vi "Path Notation to Array.vi"(11 "Item Path":string) -> (3 "Nested Item Names":string[](array[string]))   [LabVIEW 2013, in "JSONtext.lvlib"]
uses:
  JSONtext.lvlib
  support/JSONtext support.lvlib
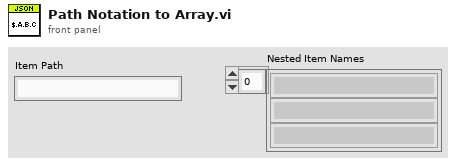
[diagram p1: front panel]
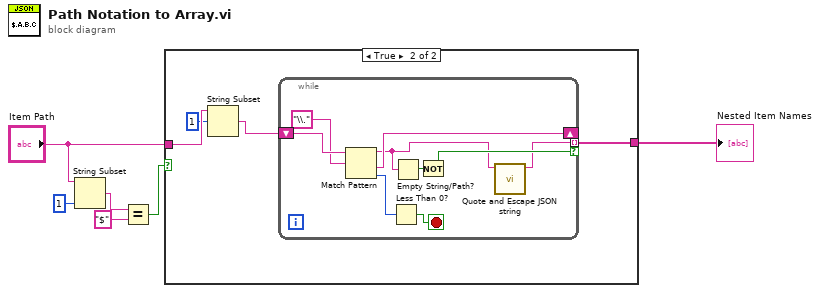
[diagram p0: block diagram]
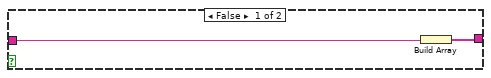
[diagram p2: hidden frame]
diagram:
  n1 = String Subset(string="Item Path", length (rest)=1 ("length (rest)")) -> (substring=w6:string)  [unwired: 1 in]
  n2 = Equal?(x=w6, y="$") -> (x = y?=w3:bool)
  n3 = case shown="True" w3 {
    tunnel: [w8 w12] -> w4
    tunnel: "Item Path" -> [w7 w11]
    frame False {
      n4 = Build Array(w7) -> (w8:string[])
    }
    frame True {
      n5 = String Subset(string=w11, offset (0)=1) -> (substring=w9:string)  [unwired: 1 in]
      n6 = while {
        tunnel: [w13] -> w12 mode=indexing if=w15
        shift-right: [w17] -> _
        shift-left: w9 -> [w21]
        stop <- w18 stop-if-true
        n7 = Match Pattern(string=w21, regular expression="\\.") -> (before substring=w14:string, after substring=w17:string, offset past match=w19:i32)  [unwired: 1 in, 1 out]
        n8 = Less Than 0?(x=w19) -> (x < 0?=w18:bool)
        n9 = Empty String/Path?(string/path=w14) -> (empty?=w16:bool)
        n10 = Not(x=w16) -> (.not. x?=w15:bool)
        n11 = call "Quote and Escape JSON string.vi"("Plain Text"=w14) -> ("<JSON>"=w13:string)  [unwired: 10 in]
      }
    }
  }
  "Nested Item Names" <- w4
